vi "Draw Feature Box.vi"(7 "Action":enum16{"Mouse Move", "Mouse Down", "Mouse Up"}(ring)=enum."Mouse Down", 8 "error in (no error)":errorcluster, 10 "UI References":T1, 11 "CtlRef":refnum<vi>) -> (0 "error out":errorcluster, 1 "Can Add?":bool, 2 "Mouse Position (Start)":cluster{"X":i32, "Y":i32})   [LabVIEW 2024]
uses:
  Controls/RVHR - UI Refs.ctl
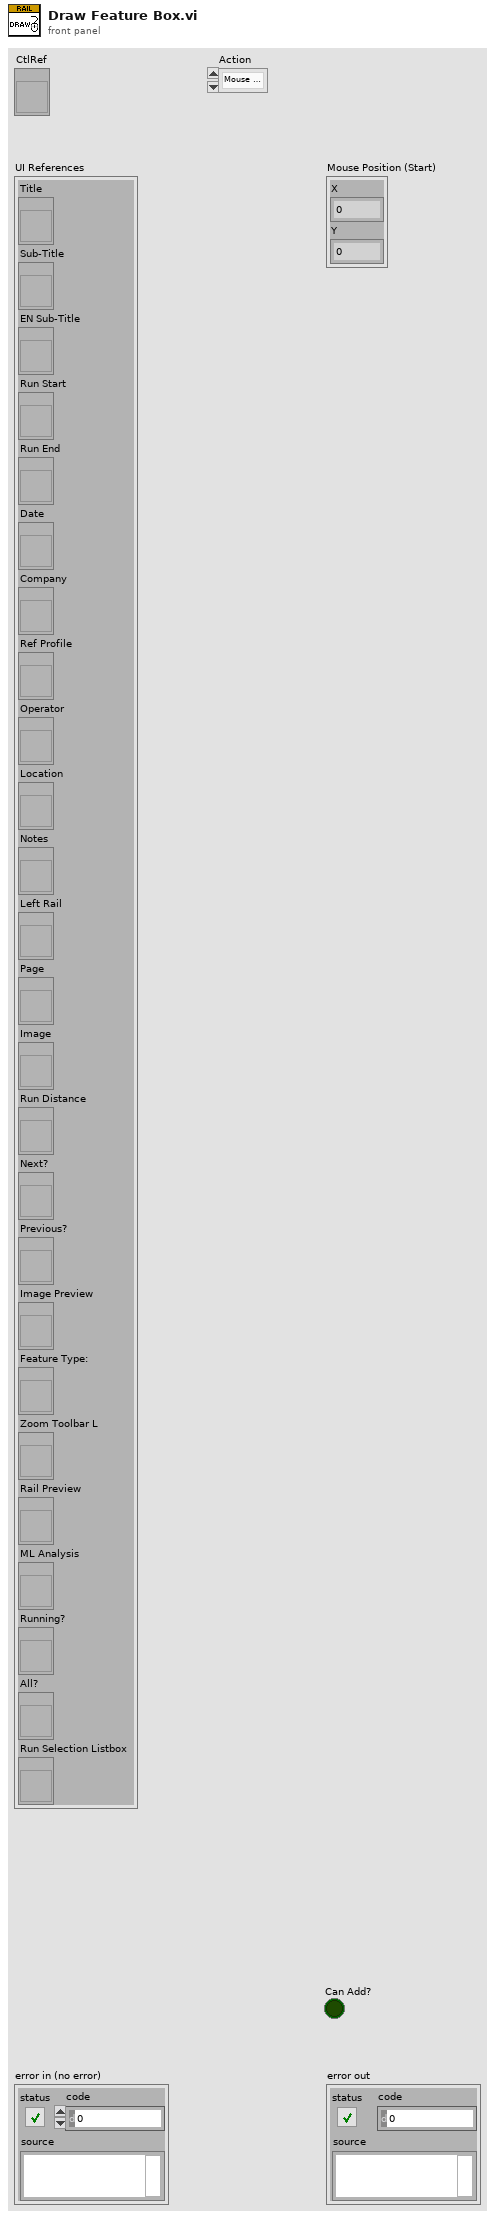
[diagram p1: front panel]
types:
  T1 = typedef "RVHR - UI Refs.ctl" = cluster{"Title":refnum<vi>, "Sub-Title":refnum<vi>, "EN Sub-Title":refnum<vi>, "Run Start":refnum<vi>, "Run End":refnum<vi>, "Date":refnum<vi>, "Company":refnum<vi>, "Ref Profile":refnum<vi>, "Operator":refnum<vi>, "Location":refnum<vi>, "Notes":refnum<vi>, "Left Rail":refnum<vi>, "Page":refnum<vi>, "Image":refnum<vi>, "Run Distance":refnum<vi>, "Next?":refnum<vi>, "Previous?":refnum<vi>, "Image Preview":refnum<vi>, "Feature Type:":refnum<vi>, "Zoom Toolbar L":refnum<vi>, "Rail Preview":refnum<vi>, "ML Analysis":refnum<vi>, "Running?":refnum<vi>, "All?":refnum<vi>, "Run Selection Listbox":refnum<vi>}
  T2 = cluster{"Width":i16, "Style":enum32{"Solid", "Dash", "Dot", "DashDot", "DashDotDot"}}
  T3 = cluster{"horizontal":enum16{"left", "center", "right"}, "vertical":enum16{"top", "center", "bottom"}}
  T4 = typedef "LVMouseTypeDef.ctl" = cluster{"Mouse Position":cluster{"X":i32, "Y":i32}, "Mouse Modifiers":cluster{"Button Down":bool, "Shift Mod":bool, "Menu Mod":bool, "Option Mod":bool}}
  T5 = cluster{"Font Name:":string, "Size":i16, "Strikeout?":bool, "Italic?":bool, "Underline?":bool, "Outline?":bool, "Shadow?":bool, "Bold?":bool}
  T6 = enum16{"User-specified Font", "Application Font", "System Font", "Dialog Font"}
  T7 = cluster{"left":i16, "top":i16, "right":i16, "bottom":i16}
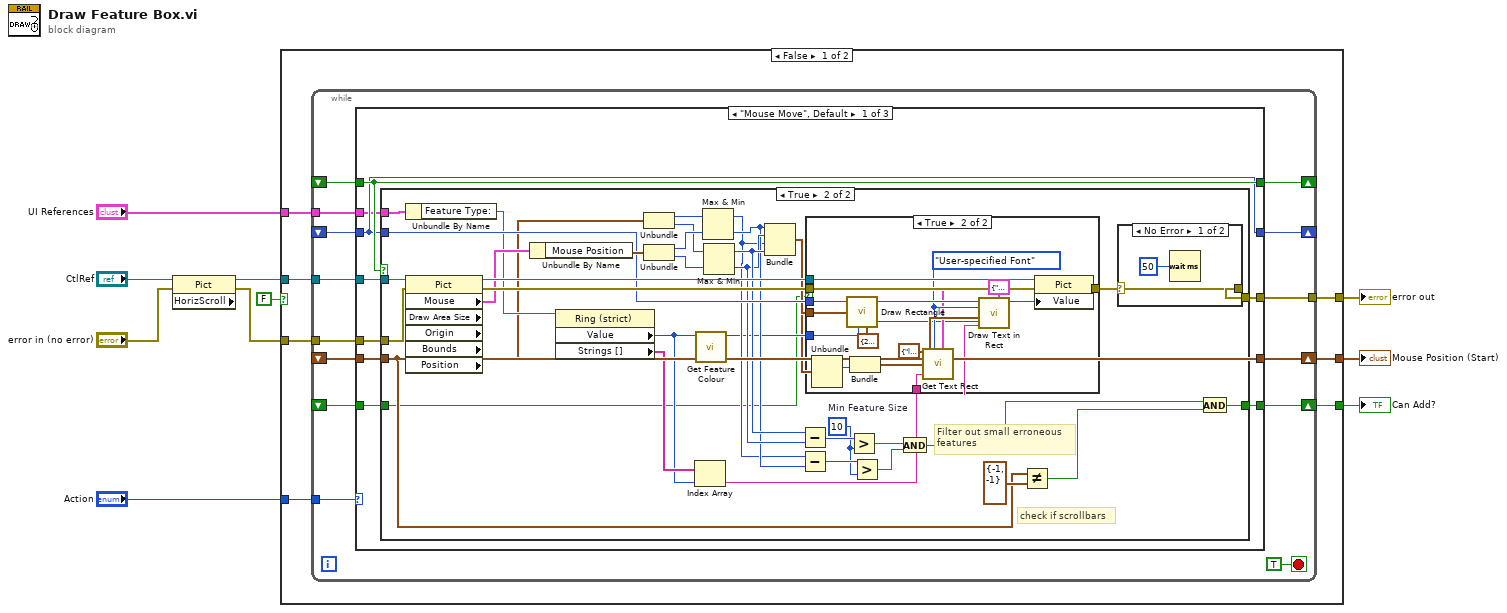
[diagram p0: block diagram]
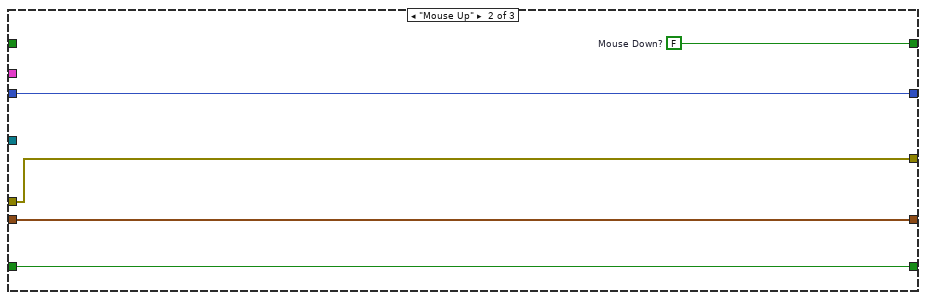
[diagram p5: hidden frame]
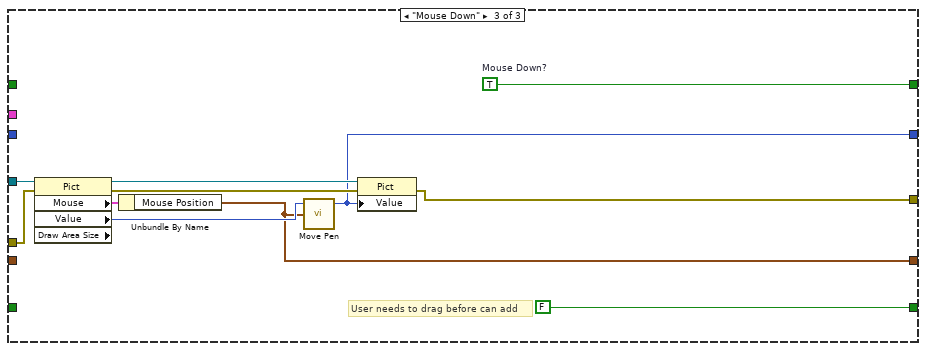
[diagram p6: hidden frame]
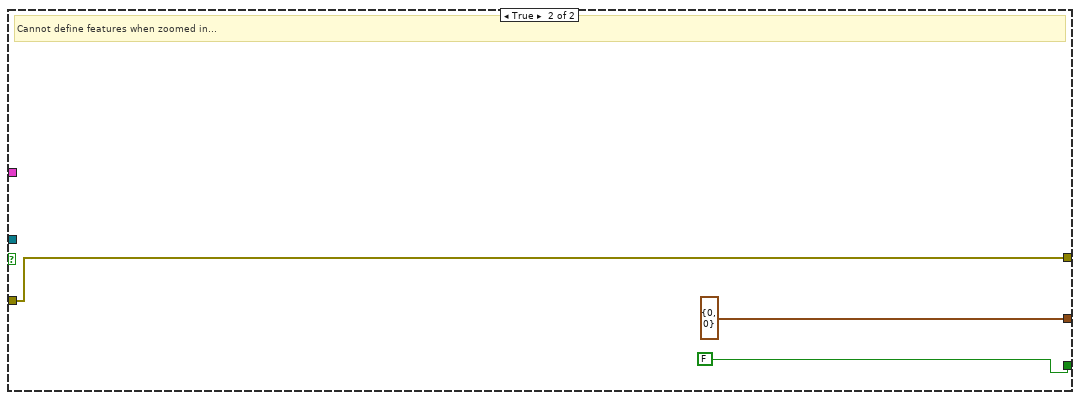
[diagram p7: hidden frame]
diagram:
  n1 = property class="Pict" props=["HorizScroll"](reference="CtlRef", error in="error in (no error)") -> (reference out=w5:refnum<vi>, error out=w3:errorcluster)  [unwired: 1 out]
  n2 = case shown="False" FALSE {
    tunnel: "Action" -> [w17 _]
    tunnel: [w16 cluster{"X":i32, "Y":i32} {"X"=0, "Y"=0} ("Mouse Position")] -> w9
    tunnel: [w15 w117] -> w7
    tunnel: "UI References" -> [w14 _]
    tunnel: w5 -> [w13 _]
    tunnel: w3 -> [w12 w117]
    tunnel: [w11 FALSE] -> w2
    frame False {
      n3 = while {
        tunnel: w17 -> [w30]
        shift-right: [w28] -> w16
        shift-left: _ -> [w29]
        tunnel: w13 -> [w27]
        tunnel: w12 -> [w26]
        tunnel: [w25] -> w15
        shift-right: [w24] -> _
        shift-left: _ -> [w23]
        shift-right: [w22] -> _
        shift-left: _ -> [w21]
        tunnel: w14 -> [w20]
        shift-right: [w19] -> w11
        shift-left: _ -> [w18]
        stop <- TRUE stop-if-true
        n4 = case shown="\"Mouse Move\", Default" w30 {
          tunnel: w29 -> [w37 w101 _]
          tunnel: [w37 w101 w104] -> w28
          tunnel: w27 -> [w40 _ w111]
          tunnel: w26 -> [w39 w102 w109]
          tunnel: [w38 w102 w108] -> w25
          tunnel: [w36 w103 w107] -> w24
          tunnel: w23 -> [w36 _ _]
          tunnel: [w35 w100 w106] -> w22
          tunnel: w21 -> [w35 w100 _]
          tunnel: w20 -> [w34 _ _]
          tunnel: [w33 w99 FALSE] -> w19
          tunnel: w18 -> [w32 w99 _]
          frame "Mouse Move", Default {
            n5 = case shown="True" w36 {
              tunnel: w40 -> [_ w69]
              tunnel: w39 -> [w42 w68]
              tunnel: [w42 w63] -> w38
              tunnel: w37 -> [_ w47]
              tunnel: w35 -> [_ w67]
              tunnel: w34 -> [_ w66]
              tunnel: [w41 w44] -> w33
              tunnel: w32 -> [w41 w43]
              frame False {
              }
              frame True {
                w56 = 10  # Min Feature Size
                # "check if scrollbars"
                # "Filter out small erroneous features"
                n6 = Unbundle By Name(w66) -> ("Feature Type:"=w65:refnum<vi>)
                n7 = property class="Pict" props=["Mouse", "Draw Area Size", "Origin", "Bounds", "Position"](reference=w69, error in=w68) -> (reference out=w71:refnum<vi>, error out=w72:errorcluster, "Mouse"=w70:T4)  [unwired: 4 out]
                n8 = Unbundle By Name(w70) -> ("Mouse Position"=w77:cluster{"X":i32, "Y":i32})
                n9 = property class="Ring (strict)"(reference=w65) -> ("Value"=w52:u16, "Strings []"=w53:string[])  [unwired: 1 in, 2 out]
                n10 = Unbundle(w47) -> ("X"=w76:i32, "Y"=w73:i32)
                n11 = Unbundle(w77) -> ("X"=w75:i32, "Y"=w74:i32)
                n12 = Index Array(array=w53, index=w52) -> (element=w51:string)
                n13 = call "Get Feature Colour.vi"("Feature Type"=w52) -> ("color"=w49:u32)  [unwired: 10 in]
                n14 = Max & Min(x=w76, y=w75) -> (max(x,y)=w59:i32, min(x,y)=w60:i32)
                n15 = Max & Min(x=w73, y=w74) -> (max(x,y)=w62:i32, min(x,y)=w61:i32)
                n16 = Bundle(w60, w61, w59, w62) -> (w50:cluster{i32, i32, i32, i32})  [unwired: 1 in]
                n17 = Subtract(x=w62, y=w61) -> (x-y=w58:i32)
                n18 = Subtract(x=w59, y=w60) -> (x-y=w57:i32)
                n19 = case shown="True" w43 {
                  tunnel: w72 -> [w78 w95]
                  tunnel: w71 -> [_ w94]
                  tunnel: w67 -> [_ w92]
                  tunnel: [w78 w91] -> w64
                  tunnel: w51 -> [_ w89]
                  tunnel: w50 -> [_ w81]
                  tunnel: w49 -> [_ w79]
                  frame False {
                  }
                  frame True {
                    w85 = T5 {"Font Name:"="Arial", "Size"=18, "Strikeout?"=FALSE, "Italic?"=FALSE, "Underline?"=FALSE, "Outline?"=FALSE, "Shadow?"=FALSE, "Bold?"=FALSE} ("[user-specified font]")
                    w86 = T6."User-specified Font" ("desired font(Application)")
                    n20 = Unbundle(w81) -> (w82:i32, w80:i32)  [unwired: 2 out]
                    n21 = call <vilib>:"Draw Rectangle.vi"("picture"=w92, "rect"=w81, "color(black)"=w79, "pen"=T2 {"Width"=2, "Style"=enum."Solid"}) -> ("new picture"=w88:picture)  [unwired: 5 in]
                    n22 = Bundle(w82, w80) -> (w83:cluster{i32, i32})  [unwired: 1 in]
                    n23 = call <vilib>:"Get Text Rect.vi"("alignment(left, top)"=T3 {"horizontal"=enum."left", "vertical"=enum."bottom"}, "desired font(Application)"=w86, "origin(0,0)"=w83, "text"=w89, "[user-specified font]"=w85) -> ("rect"=w90:T7)  [unwired: 4 in]
                    n24 = call <vilib>:"Draw Text in Rect.vi"("[user-specified font]"=w85, "text color(black)"=w79, "desired font(Application)"=w86, "text"=w89, "rect"=w90, "picture"=w88) -> ("new picture"=w87:picture)  [unwired: 5 in]
                    n25 = property class="Pict"(reference=w94, error in=w95, "Value"=w87) -> (error out=w91:errorcluster)  [unwired: 1 out]
                  }
                }
                n26 = Greater?(x=w58, y=w56) -> (0:w55:bool)
                n27 = Greater?(x=w57, y=w56) -> (0:w54:bool)
                n28 = And(x=w55, y=w54) -> (x .and. y?=w46:bool)
                n29 = Not Equal?(x=w47, y=cluster{"X":i32, "Y":i32} {"X"=-1, "Y"=-1} ("Mouse Position")) -> (x != y?=w45:bool)
                n30 = case shown="No Error" w64 {
                  selector: w64 -> [w97 w98]
                  tunnel: [w97 w98] -> w63
                  frame No Error {
                    n31 = Wait (ms)(milliseconds to wait=u32 50) -> ()  [unwired: 1 out]
                  }
                  frame Error {
                  }
                }
                n32 = And(x=w46, y=w45) -> (x .and. y?=w44:bool)
              }
            }
          }
          frame "Mouse Up" {
            w103 = FALSE  # Mouse Down?
          }
          frame "Mouse Down" {
            w107 = TRUE  # Mouse Down?
            # "User needs to drag before can add"
            n33 = property class="Pict" props=["Mouse", "Value", "Draw Area Size"](reference=w111, error in=w109) -> (reference out=w110:refnum<vi>, error out=w114:errorcluster, "Mouse"=w112:T4, "Value"=w113:picture)  [unwired: 1 out]
            n34 = Unbundle By Name(w112) -> ("Mouse Position"=w104:cluster{"X":i32, "Y":i32})
            n35 = call <vilib>:"Move Pen.vi"("new position"=w104, "picture"=w113) -> ("new picture"=w106:picture)  [unwired: 3 in]
            n36 = property class="Pict"(reference=w110, error in=w114, "Value"=w106) -> (error out=w108:errorcluster)  [unwired: 1 out]
          }
        }
      }
    }
    frame True {
      # "Cannot define features when zoomed in..."
    }
  }
  "Mouse Position (Start)" <- w9
  "error out" <- w7
  "Can Add?" <- w2
